vi "Decode PDO.vi"() -> ()   [LabVIEW 2016]
uses:
  <vilib>/CANopenLib/CANOPEN.llb/CANopen TPDO Create.vi
  <vilib>/CANopenLib/CANOPEN.llb/CANopen TPDO Start.vi
  <vilib>/CANopenLib/CANOPEN.llb/CANopen TPDO Stop.vi
  <vilib>/CANopenLib/CANOPEN.llb/CANopen TPDO Close.vi
panel:
  out "data 4":u8[](array[numeric])
  out "data 3":u8[](array[numeric])
  out "data 2":u8[](array[numeric])
  out "data":u8[](array[numeric])
  out "error out":errorcluster
  in  "Motor":u8(ring) items=["Right", "Left"]
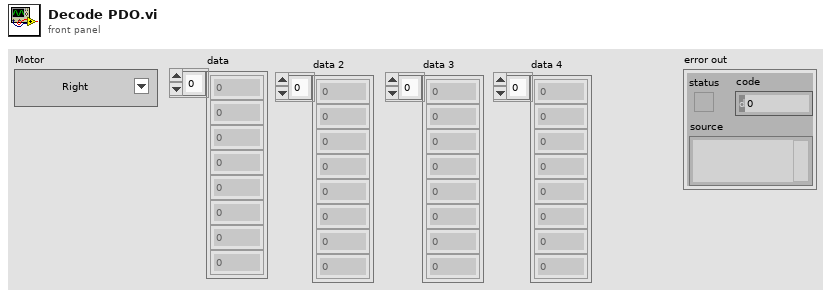
[diagram p1: front panel]
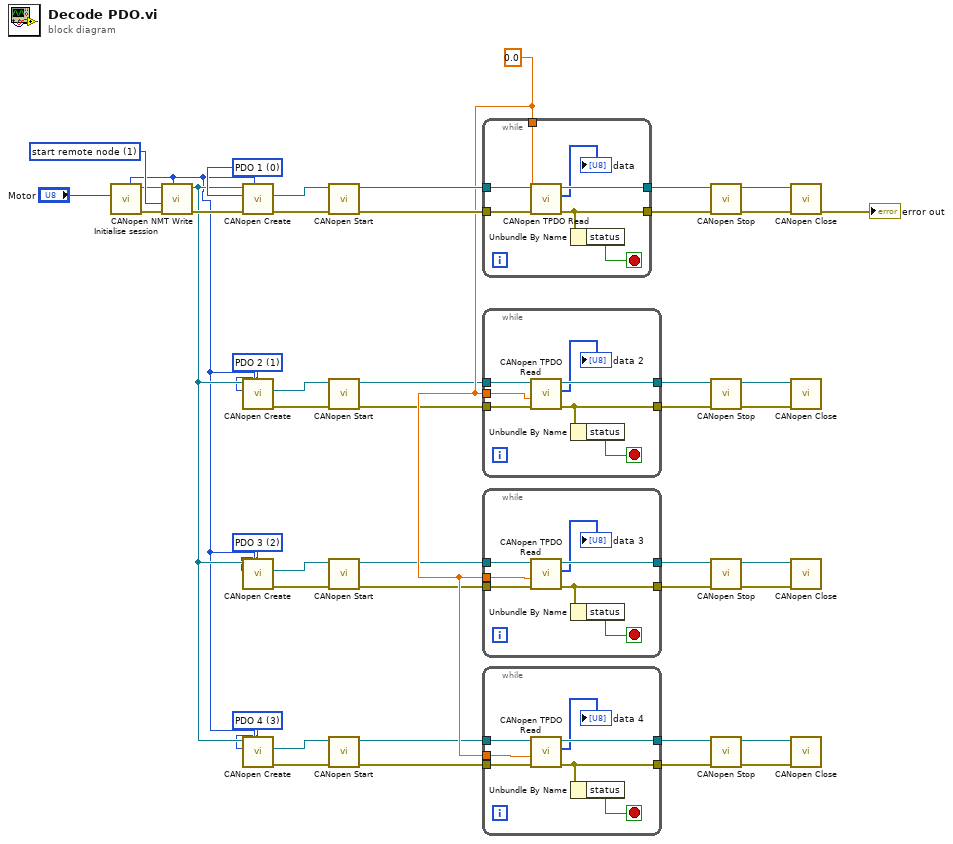
[diagram p0: block diagram]
diagram:
  w1 = u8 3 items=["PDO 1", "PDO 2", "PDO 3", "PDO 4"] ("PDO channel")
  w2 = u8 2 items=["PDO 1", "PDO 2", "PDO 3", "PDO 4"] ("PDO channel")
  w3 = u8 1 items=["PDO 1", "PDO 2", "PDO 3", "PDO 4"] ("PDO channel")
  w34 = u16 1 items=["start remote node"=1, "stop remote node"=2, "enter pre-operational"=128, "reset node"=129, "reset communication"=130] ("command")
  w28 = 0.0 ("timeout (0s)")
  w36 = u8 0 items=["PDO 1", "PDO 2", "PDO 3", "PDO 4"] ("PDO channel")
  n1 = call "Initialise session.vi"("Motor"="Motor") -> ("error out"=w31:errorcluster, "interface object out"=w33:refnum<k20>, "Used Node ID"=w29:u8)  [unwired: 8 in]
  n2 = call <vilib>:"CANopen NMT Write.vi"("node-ID (0)"=w29, "error in (no error)"=w31, "command"=w34, "interface object in"=w33) -> ("error out"=w32:errorcluster, "interface object out"=w30:refnum<k20>)  [unwired: 6 in]
  n3 = call-poly <vilib>:"CANopen Create.vi"("node-ID"=w29, "error in (no error)"=w32, "PDO channel"=w36, "interface object in"=w30) -> ("error out"=w45:errorcluster, "TPDO object out"=w44:refnum<k20>)  [unwired: 5 in, 1 out]
  n4 = call-poly <vilib>:"CANopen Create.vi"("node-ID"=w29, "PDO channel"=w3, "interface object in"=w30) -> ("error out"=w20:errorcluster, "TPDO object out"=w21:refnum<k20>)  [unwired: 6 in, 1 out]
  n5 = call-poly <vilib>:"CANopen Create.vi"("node-ID"=w29, "PDO channel"=w2, "interface object in"=w30) -> ("error out"=w19:errorcluster, "TPDO object out"=w18:refnum<k20>)  [unwired: 6 in, 1 out]
  n6 = call-poly <vilib>:"CANopen Create.vi"("node-ID"=w29, "PDO channel"=w1, "interface object in"=w30) -> ("error out"=w4:errorcluster, "TPDO object out"=w5:refnum<k20>)  [unwired: 6 in, 1 out]
  n7 = call-poly <vilib>:"CANopen Start.vi"("error in (no error)"=w45, "TPDO object in"=w44) -> ("error out"=w42:errorcluster, "TPDO object out"=w43:refnum<k20>)  [unwired: 8 in]
  n8 = call-poly <vilib>:"CANopen Start.vi"("error in (no error)"=w20, "TPDO object in"=w21) -> ("error out"=w23:errorcluster, "TPDO object out"=w22:refnum<k20>)  [unwired: 8 in]
  n9 = call-poly <vilib>:"CANopen Start.vi"("error in (no error)"=w19, "TPDO object in"=w18) -> ("error out"=w16:errorcluster, "TPDO object out"=w17:refnum<k20>)  [unwired: 8 in]
  n10 = call-poly <vilib>:"CANopen Start.vi"("error in (no error)"=w4, "TPDO object in"=w5) -> ("error out"=w7:errorcluster, "TPDO object out"=w6:refnum<k20>)  [unwired: 8 in]
  n11 = while {
    tunnel: w28 -> [w48]
    tunnel: w42 -> [w51]
    tunnel: [w47] -> w40
    tunnel: w43 -> [w52]
    tunnel: [w50] -> w41
    stop <- w46 stop-if-true
    n12 = call <vilib>:"CANopen TPDO Read.vi"("error in (no error)"=w51, "timeout (0s)"=w48, "TPDO object in"=w52) -> ("error out"=w47:errorcluster, "data"=→"data":u8[], "TPDO object out"=w50:refnum<k20>)  [unwired: 4 in, 2 out]
    n13 = Unbundle By Name(w47) -> ("status"=w46:bool)
  }
  n14 = while {
    tunnel: w23 -> [w58]
    tunnel: [w55] -> w25
    tunnel: w22 -> [w59]
    tunnel: [w57] -> w24
    tunnel: w28 -> [w53]
    stop <- w54 stop-if-true
    n15 = call <vilib>:"CANopen TPDO Read.vi"("error in (no error)"=w58, "timeout (0s)"=w53, "TPDO object in"=w59) -> ("error out"=w55:errorcluster, "data"=→"data 2":u8[], "TPDO object out"=w57:refnum<k20>)  [unwired: 4 in, 2 out]
    n16 = Unbundle By Name(w55) -> ("status"=w54:bool)
  }
  n17 = while {
    tunnel: w16 -> [w65]
    tunnel: [w62] -> w14
    tunnel: w17 -> [w66]
    tunnel: [w64] -> w15
    tunnel: w28 -> [w60]
    stop <- w61 stop-if-true
    n18 = call <vilib>:"CANopen TPDO Read.vi"("error in (no error)"=w65, "timeout (0s)"=w60, "TPDO object in"=w66) -> ("error out"=w62:errorcluster, "data"=→"data 3":u8[], "TPDO object out"=w64:refnum<k20>)  [unwired: 4 in, 2 out]
    n19 = Unbundle By Name(w62) -> ("status"=w61:bool)
  }
  n20 = while {
    tunnel: w7 -> [w72]
    tunnel: [w69] -> w9
    tunnel: w6 -> [w73]
    tunnel: [w71] -> w8
    tunnel: w28 -> [w67]
    stop <- w68 stop-if-true
    n21 = call <vilib>:"CANopen TPDO Read.vi"("error in (no error)"=w72, "timeout (0s)"=w67, "TPDO object in"=w73) -> ("error out"=w69:errorcluster, "data"=→"data 4":u8[], "TPDO object out"=w71:refnum<k20>)  [unwired: 4 in, 2 out]
    n22 = Unbundle By Name(w69) -> ("status"=w68:bool)
  }
  n23 = call-poly <vilib>:"CANopen Stop.vi"("error in (no error)"=w40, "TPDO object in"=w41) -> ("error out"=w38:errorcluster, "TPDO object out"=w39:refnum<k20>)  [unwired: 8 in]
  n24 = call-poly <vilib>:"CANopen Stop.vi"("error in (no error)"=w25, "TPDO object in"=w24) -> ("error out"=w27:errorcluster, "TPDO object out"=w26:refnum<k20>)  [unwired: 8 in]
  n25 = call-poly <vilib>:"CANopen Stop.vi"("error in (no error)"=w14, "TPDO object in"=w15) -> ("error out"=w12:errorcluster, "TPDO object out"=w13:refnum<k20>)  [unwired: 8 in]
  n26 = call-poly <vilib>:"CANopen Stop.vi"("error in (no error)"=w9, "TPDO object in"=w8) -> ("error out"=w11:errorcluster, "TPDO object out"=w10:refnum<k20>)  [unwired: 8 in]
  n27 = call-poly <vilib>:"CANopen Close.vi"("error in (no error)"=w38, "TPDO object in"=w39) -> ("error out"=→"error out":errorcluster)  [unwired: 9 in]
  n28 = call-poly <vilib>:"CANopen Close.vi"("error in (no error)"=w27, "TPDO object in"=w26) -> ()  [unwired: 9 in, 1 out]
  n29 = call-poly <vilib>:"CANopen Close.vi"("error in (no error)"=w12, "TPDO object in"=w13) -> ()  [unwired: 9 in, 1 out]
  n30 = call-poly <vilib>:"CANopen Close.vi"("error in (no error)"=w11, "TPDO object in"=w10) -> ()  [unwired: 9 in, 1 out]
